vi "time_array_3.vi"() -> ()   [LabVIEW 2017]
panel:
  out "最近五筆大於0.9":dbl[][](array[numeric])
  out "最近五筆小於0.9":dbl[][](array[numeric])
  out "最新十筆":dbl[][](array[numeric])
  out "控制指示燈":bool
  in  "迴圈速率":u32
  out "最新數據":dbl[](array[numeric])
  out "day":dbl(knob) scale=0.0..10.0
  out "hr":dbl(knob) scale=0.0..10.0
  out "min":dbl(knob) scale=0.0..60.0
  out "迴圈次數":i32
  in  "stop":bool
  out "s":dbl(knob) scale=0.0..60.0
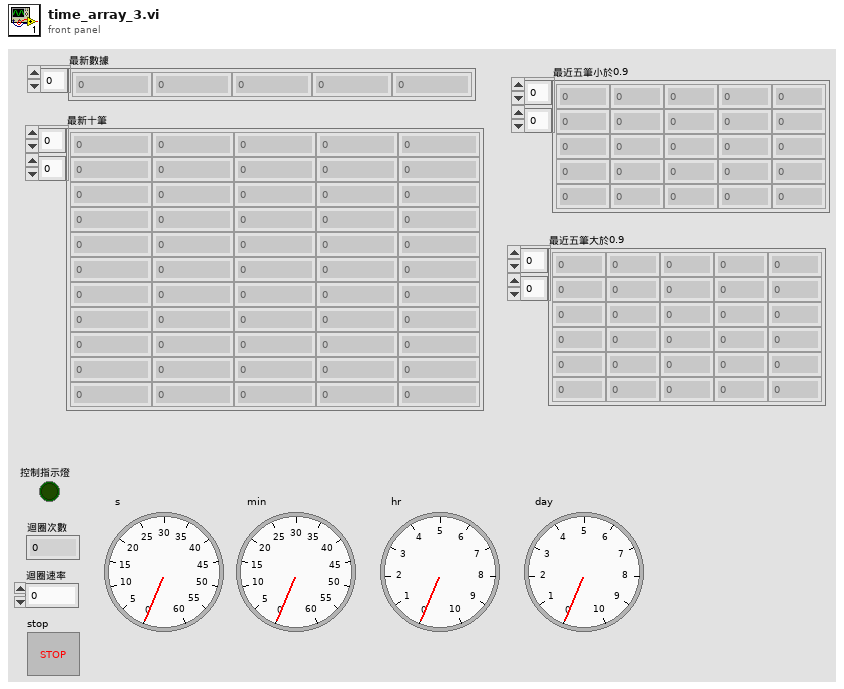
[diagram p1: front panel]
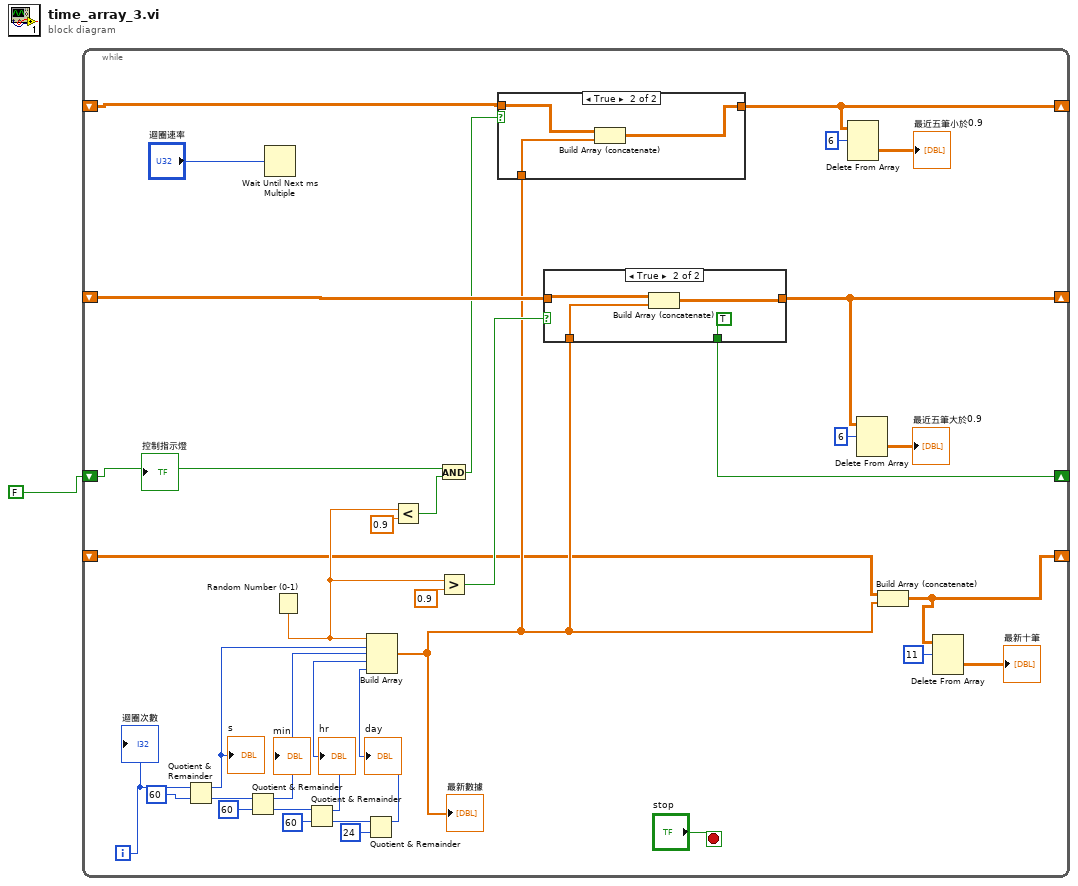
[diagram p0: block diagram]
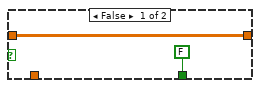
[diagram p3: hidden frame]
diagram:
  n1 = while {
    shift-right: [w3] -> _
    shift-left: _ -> [w21]
    shift-right: [w20] -> _
    shift-left: FALSE -> [w16]
    shift-right: [w2] -> _
    shift-left: _ -> [w13]
    shift-right: [w9] -> _
    shift-left: _ -> [w10]
    i -> [w35]
    stop <- "stop" stop-if-true
    n2 = Quotient & Remainder(x=w35, y=60) -> (x-y*floor(x/y)=w27:i32, floor(x/y)=w33:i32)
    "s" <- w27
    n3 = Quotient & Remainder(x=w33, y=60) -> (x-y*floor(x/y)=w26:i32, floor(x/y)=w31:i32)
    "min" <- w26
    n4 = Wait Until Next ms Multiple(millisecond multiple="迴圈速率") -> ()  [unwired: 1 out]
    n5 = Random Number (0-1)() -> (number: 0 to 1=w17:dbl)
    n6 = Quotient & Remainder(x=w31, y=60) -> (x-y*floor(x/y)=w25:i32, floor(x/y)=w29:i32)
    "hr" <- w25
    n7 = Quotient & Remainder(x=w29, y=24) -> (x-y*floor(x/y)=w24:i32)  [unwired: 1 out]
    "day" <- w24
    n8 = Build Array(w17, w27, w26, w25, w24) -> (w11:dbl[])
    "最新數據" <- w11
    n9 = Less?(x=w17, y=0.9) -> (x < y?=w15:bool)
    n10 = And(x=w16, y=w15) -> (x .and. y?=w14:bool)
    n11 = Greater?(x=w17, y=0.9) -> (0:w19:bool)
    n12 = case shown="True" w14 {
      tunnel: w13 -> [w37 w40]
      tunnel: [w37 w38] -> w2
      tunnel: w11 -> [_ w39]
      frame False {
      }
      frame True {
        n13 = Build Array (concatenate)(w40, w39) -> (w38:dbl[][])
      }
    }
    n14 = case shown="True" w19 {
      tunnel: w11 -> [_ w44]
      tunnel: w21 -> [w41 w46]
      tunnel: [w41 w43] -> w3
      tunnel: [FALSE TRUE] -> w20
      frame False {
      }
      frame True {
        n15 = Build Array (concatenate)(w46, w44) -> (w43:dbl[][])
      }
    }
    n16 = Delete From Array(array=w2, length=6) -> (deleted portion=→"最近五筆小於0.9":dbl[][])  [unwired: 2 in, 1 out]
    n17 = Delete From Array(array=w3, length=6) -> (deleted portion=→"最近五筆大於0.9":dbl[][])  [unwired: 2 in, 1 out]
    n18 = Build Array (concatenate)(w10, w11) -> (w9:dbl[][])
    n19 = Delete From Array(array=w9, length=11) -> (deleted portion=→"最新十筆":dbl[][])  [unwired: 2 in, 1 out]
    "迴圈次數" <- w35
    "控制指示燈" <- w16
  }
